vi "check if within max permissible voltage range.vi"(8 "error in (no error)":errorcluster, 11 "ImagingModeSPIM in":refnum<class "ImagingModeSPIM.lvclass">) -> (0 "error out":errorcluster, 3 "ImagingModeSPIM out":refnum<class "ImagingModeSPIM.lvclass">)   [LabVIEW 2012]
uses:
  ImagingModeSPIM.lvclass
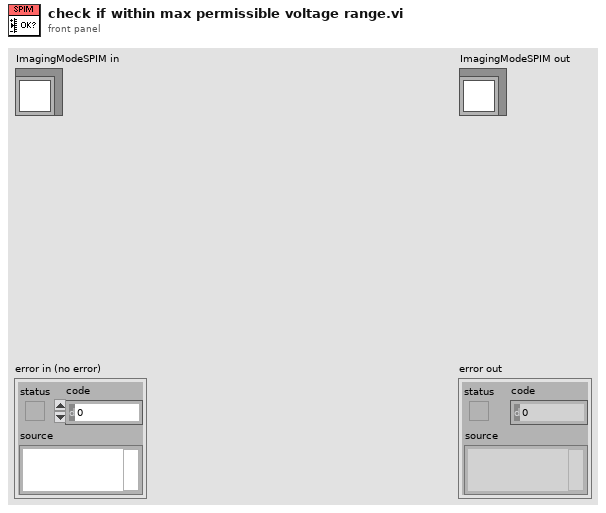
[diagram p1: front panel]
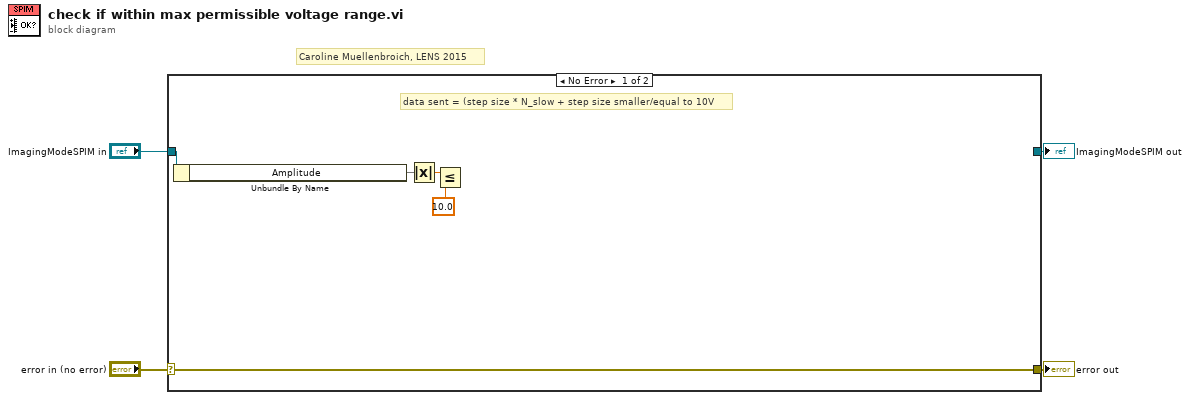
[diagram p0: block diagram]
diagram:
  # "Caroline Muellenbroich, LENS 2015"
  n1 = case shown="No Error" "error in (no error)" {
    selector: "error in (no error)" -> [w10 w12]
    tunnel: [w10 w12] -> w3
    tunnel: [_ w11] -> w1
    tunnel: "ImagingModeSPIM in" -> [w5 w11]
    frame No Error {
      # "data sent = (step size * N_slow + step size smaller/equal to 10V"
      n2 = Unbundle By Name(w5) -> ("Amplitude"=w8)
      n3 = Absolute Value(x=w8) -> (abs(x)=w9:dbl)
      n4 = Less Or Equal?(x=w9, y=dbl[unit] 10.0) -> (x <= y?=w6:bool)
    }
    frame Error {
    }
  }
  "error out" <- w3
  "ImagingModeSPIM out" <- w1
